vi "HumanTrajPositions.vi"(10 "FieldPos":T1(ring), 11 "Init":bool) -> (1 "vAngular":dbl, 2 "vY":dbl, 3 "vX":dbl)   [LabVIEW 2023]
uses:
  <vilib>/Rock Robotics/WPI/ThirdParty/JAS_Junk/TrajLib/Rotation2d_CreateAngle.vi
  <vilib>/Rock Robotics/WPI/ThirdParty/JAS_Junk/TrajLib/Translation2d_Create.vi
  <vilib>/Rock Robotics/WPI/ThirdParty/JAS_Junk/TrajLib/Trajectory_Library.lvlib
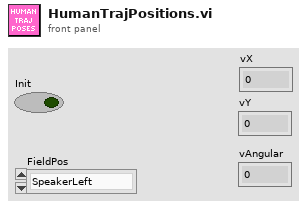
[diagram p1: front panel]
types:
  T1 = enum16{"SpeakerLeft", "SpeakerCenter", "SpeakerRight", "Amp", "Source", "StageLeft", "StageCenter", "StageRight"}
  T2 = typedef "WPI_DriverStationAllianceInfo.ctl" = enum16{"Red", "Blue", "Invalid"}
  T3 = typedef "Trajectory_Library.lvlib/POSE2D.ctl" = cluster{"TRANSLATION":T4, "ROTATION":T5}
  T4 = typedef "Trajectory_Library.lvlib/TRANSLATION2D.ctl" = cluster{"X":dbl, "Y":dbl}
  T5 = typedef "Trajectory_Library.lvlib/ROTATION2D.ctl" = cluster{"VALUE":dbl, "COS":dbl, "SIN":dbl}
  T6 = typedef "Trajectory_Library.lvlib/CHASSIS_SPEEDS.ctl" = cluster{"vX":dbl, "vY":dbl, "vOmega":dbl}
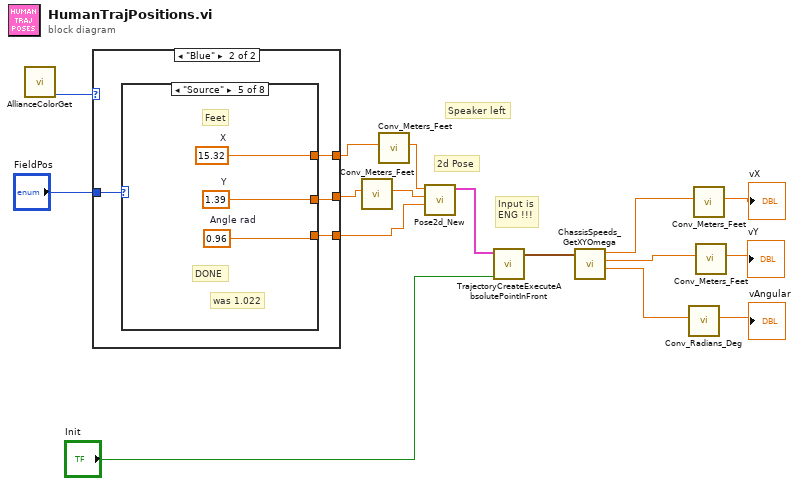
[diagram p0: block diagram]
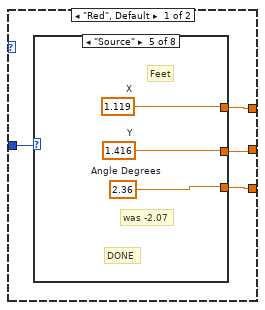
[diagram p2: hidden frame]
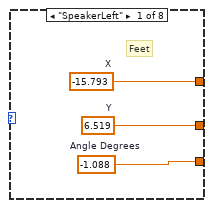
[diagram p3: hidden frame]
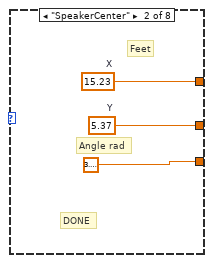
[diagram p4: hidden frame]
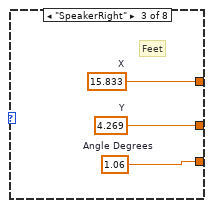
[diagram p5: hidden frame]
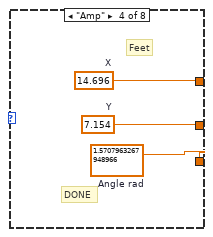
[diagram p6: hidden frame]
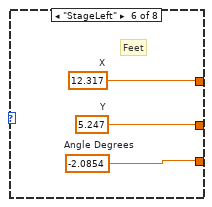
[diagram p7: hidden frame]
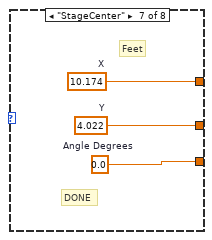
[diagram p8: hidden frame]
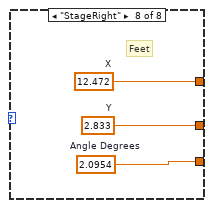
[diagram p9: hidden frame]
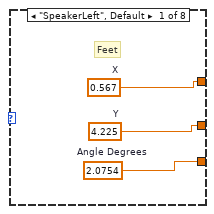
[diagram p10: hidden frame]
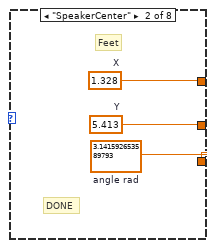
[diagram p11: hidden frame]
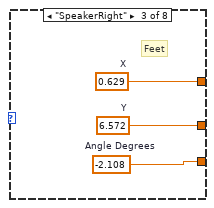
[diagram p12: hidden frame]
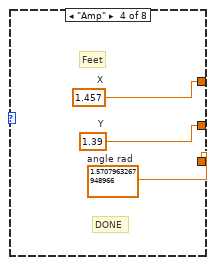
[diagram p13: hidden frame]
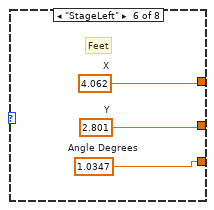
[diagram p14: hidden frame]
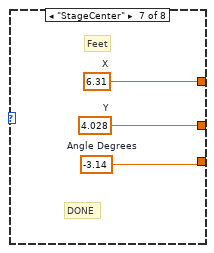
[diagram p15: hidden frame]
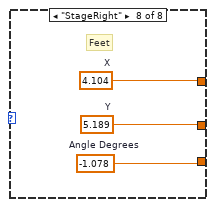
[diagram p16: hidden frame]
diagram:
  # "Input is\nENG !!!"
  # "2d Pose"
  # "Speaker left"
  n1 = call "AllianceColorGet.vi"() -> ("AllianceColor"=w12:T2)  [unwired: 11 in]
  n2 = case shown="\"Blue\"" w12 {
    tunnel: [w18 w48] -> w11
    tunnel: [w19 w47] -> w8
    tunnel: [w20 w46] -> w10
    tunnel: "FieldPos" -> [w17 w45]
    frame "Red", Default {
      n3 = case shown="\"Source\"" w17 {
        tunnel: [w21 3.141592653589793 w29 w30 w33 w36 w39 w44] -> w18
        tunnel: [w22 w25 w28 w31 w34 w37 w40 w43] -> w19
        tunnel: [w23 w26 w27 w32 w35 w38 w41 w42] -> w20
        frame "SpeakerLeft" {
          w23 = -15.793  # X
          w22 = 6.519  # Y
          w21 = -1.088  # Angle Degrees
          # "Feet"
        }
        frame "SpeakerCenter" {
          w26 = 15.23  # X
          w25 = 5.37  # Y
          # "DONE"
          # "Angle rad"
          # "Feet"
        }
        frame "SpeakerRight" {
          w27 = 15.833  # X
          w28 = 4.269  # Y
          w29 = 1.06  # Angle Degrees
          # "Feet"
        }
        frame "Amp" {
          w30 = 1.5707963267948966  # Angle rad
          w32 = 14.696  # X
          w31 = 7.154  # Y
          # "DONE"
          # "Feet"
        }
        frame "Source" {
          w35 = 1.119  # X
          w34 = 1.416  # Y
          w33 = 2.36  # Angle Degrees
          # "DONE"
          # "was -2.07"
          # "Feet"
        }
        frame "StageLeft" {
          w38 = 12.317  # X
          w37 = 5.247  # Y
          w36 = -2.0854  # Angle Degrees
          # "Feet"
        }
        frame "StageCenter" {
          w41 = 10.174  # X
          w40 = 4.022  # Y
          w39 = 0.0  # Angle Degrees
          # "DONE"
          # "Feet"
        }
        frame "StageRight" {
          w42 = 12.472  # X
          w43 = 2.833  # Y
          w44 = 2.0954  # Angle Degrees
          # "Feet"
        }
      }
    }
    frame "Blue" {
      n4 = case shown="\"Source\"" w45 {
        tunnel: [w49 w52 w57 w58 w61 w64 w67 w70] -> w48
        tunnel: [w50 w53 w56 w59 w62 w65 w68 w71] -> w47
        tunnel: [w51 w54 w55 w60 w63 w66 w69 w72] -> w46
        frame "SpeakerLeft", Default {
          w51 = 0.567  # X
          w50 = 4.225  # Y
          w49 = 2.0754  # Angle Degrees
          # "Feet"
        }
        frame "SpeakerCenter" {
          w52 = 3.141592653589793  # angle rad
          w54 = 1.328  # X
          w53 = 5.413  # Y
          # "DONE"
          # "Feet"
        }
        frame "SpeakerRight" {
          w55 = 0.629  # X
          w56 = 6.572  # Y
          w57 = -2.108  # Angle Degrees
          # "Feet"
        }
        frame "Amp" {
          w58 = 1.5707963267948966  # angle rad
          w60 = 1.457  # X
          w59 = 1.39  # Y
          # "DONE"
          # "Feet"
        }
        frame "Source" {
          w63 = 15.32  # X
          w62 = 1.39  # Y
          w61 = 0.96  # Angle rad
          # "DONE"
          # "was 1.022"
          # "Feet"
        }
        frame "StageLeft" {
          w66 = 4.062  # X
          w65 = 2.801  # Y
          w64 = 1.0347  # Angle Degrees
          # "Feet"
        }
        frame "StageCenter" {
          w69 = 6.31  # X
          w68 = 4.028  # Y
          w67 = -3.14  # Angle Degrees
          # "DONE"
          # "Feet"
        }
        frame "StageRight" {
          w72 = 4.104  # X
          w71 = 5.189  # Y
          w70 = -1.078  # Angle Degrees
          # "Feet"
        }
      }
    }
  }
  n5 = call <vilib>:"Conv_Meters_Feet.vi"("Meters"=w8) -> ("Feet"=w7:dbl)  [unwired: 10 in]
  n6 = call <vilib>:"Conv_Meters_Feet.vi"("Meters"=w10) -> ("Feet"=w9:dbl)  [unwired: 10 in]
  n7 = call <vilib>:"Pose2d_New.vi"("Heading"=w11, "Y"=w7, "X"=w9) -> ("out POSe"=w16:T3)  [unwired: 8 in]
  n8 = call "TrajectoryCreateExecuteAbsolutePointInFront.vi"("Init"="Init", "End Pose ENG"=w16) -> ("Chassis Velocity Target"=w15:T6)  [unwired: 8 in, 1 out]
  n9 = call <vilib>:"ChassisSpeeds_GetXYOmega.vi"("CHASSIS"=w15) -> ("vAngular"=w1:dbl, "vY"=w5:dbl, "vX"=w6:dbl)  [unwired: 8 in]
  n10 = call <vilib>:"Conv_Radians_Deg.vi"("Radians"=w1) -> ("Degrees"=→"vAngular":dbl)  [unwired: 10 in]
  n11 = call <vilib>:"Conv_Meters_Feet.vi"("Meters"=w6) -> ("Feet"=→"vX":dbl)  [unwired: 10 in]
  n12 = call <vilib>:"Conv_Meters_Feet.vi"("Meters"=w5) -> ("Feet"=→"vY":dbl)  [unwired: 10 in]
